vi "Gyro Open.vi"(11 "refnum name":string="Ye Newe Gyro") -> (0 "error out":errorcluster, 3 "I2CDevRef":T1={"DevStatus"={"status"=FALSE, "code"=0, "source"=""}, "Device Address"=0, "Handle"=0, "I2C Bus"=enum."Invalid"} {"Device Address" format="%.0x"})   [LabVIEW 2015]
uses:
  <vilib>/Rock Robotics/WPI/I2C/WPI_I2CDevRef.ctl
  <vilib>/Rock Robotics/SystemInterfaces/i2clib/i2c_bus.ctl
panel:
  out "Data Out":u8[](array[numeric])
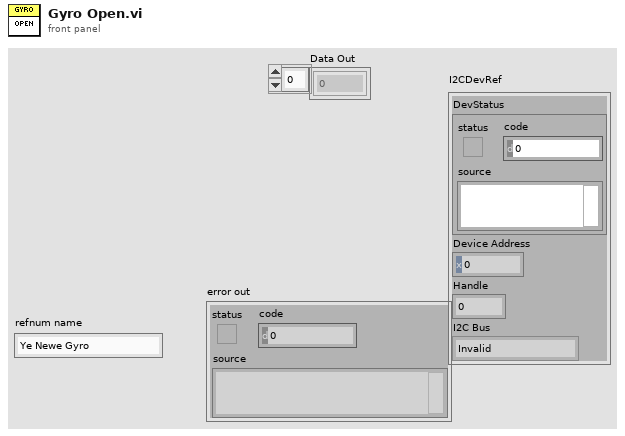
[diagram p1: front panel]
types:
  T1 = typedef "WPI_I2CDevRef.ctl" = cluster{"DevStatus":errorcluster, "Device Address":u8, "Handle":i32, "I2C Bus":T2}
  T2 = typedef "i2c_bus.ctl" = enum16{"I2C On-Board", "I2C MXP", "Invalid"}
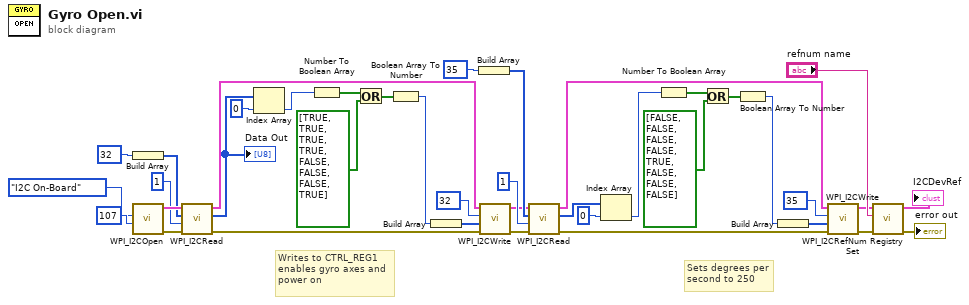
[diagram p0: block diagram]
diagram:
  # "Sets degrees per\nsecond to 250"
  # "Writes to CTRL_REG1\nenables gyro axes and\npower on"
  n1 = Build Array(u8 32 ("Data To Send")) -> (w35:u8[])
  n2 = call <vilib>:"WPI_I2COpen.vi"("Device Address"=u8 107 ("Data To Send"), "I2C Bus"=i2c_bus."I2C On-Board") -> ("error out"=w2:errorcluster, "I2CDevRef"=w37:T1)  [unwired: 8 in]
  n3 = call <vilib>:"WPI_I2CRead.vi"("error in (no error)"=w2, "I2CBytesToRead"=u8 1, "I2CRegister"=w35, "I2CDevRef"=w37) -> ("error out"=w25:errorcluster, "Data Out"=w33:u8[], "I2CDevRef"=w24:T1)  [unwired: 5 in]
  "Data Out" <- w33
  n4 = Index Array(array=w33, index=0) -> (element=w31:u8)
  n5 = Number To Boolean Array(number=w31) -> (Boolean array=w29:bool[])
  n6 = Or(x=w29, y=bool[] [TRUE, TRUE, TRUE, TRUE, FALSE, FALSE, FALSE, TRUE] ("Boolean array")) -> (x .or. y?=w28:bool[])
  n7 = Boolean Array To Number(Boolean array=w28) -> (number=w27:u32)
  n8 = Build Array(w27) -> (w26:u32[])
  n9 = Build Array(u8 35 ("Data To Send")) -> (w11:u8[])
  n10 = call <vilib>:"WPI_I2CWrite.vi"("error in (no error)"=w25, "I2CDataToSend"=w26, "I2CRegister"=u8 32 ("Data To Send"), "I2CDevRef"=w24) -> ("error out"=w5:errorcluster, "I2CDevRef"=w6:T1)  [unwired: 6 in]
  n11 = call <vilib>:"WPI_I2CRead.vi"("error in (no error)"=w5, "I2CBytesToRead"=u8 1, "I2CRegister"=w11, "I2CDevRef"=w6) -> ("error out"=w15:errorcluster, "Data Out"=w21:u8[], "I2CDevRef"=w16:T1)  [unwired: 5 in]
  n12 = Index Array(array=w21, index=0) -> (element=w19:u8)
  n13 = Number To Boolean Array(number=w19) -> (Boolean array=w20:bool[])
  n14 = Or(x=w20, y=bool[] [FALSE, FALSE, FALSE, FALSE, TRUE, FALSE, FALSE, FALSE] ("Boolean array")) -> (x .or. y?=w17:bool[])
  n15 = Boolean Array To Number(Boolean array=w17) -> (number=w14:u32)
  n16 = Build Array(w14) -> (w13:u32[])
  n17 = call <vilib>:"WPI_I2CWrite.vi"("error in (no error)"=w15, "I2CDataToSend"=w13, "I2CRegister"=u8 35 ("Data To Send"), "I2CDevRef"=w16) -> ("error out"=w8:errorcluster, "I2CDevRef"=w9:T1)  [unwired: 6 in]
  n18 = call <vilib>:"WPI_I2CRefNum Registry Set.vi"("error in (no error)"=w8, "refnum name"="refnum name", "I2CDevRef"=w9) -> ("error out"=→"error out":errorcluster, "I2CDevRef"=→"I2CDevRef":T1)  [unwired: 7 in]
